vi "PID_controller_14.vi"() -> ()   [LabVIEW 2011]
panel:
  in  "Tune":bool
  out "Temp Set Point (torr)":dbl
  in  "stop":bool
  out "fit":cluster{"element":dbl, "Value":dbl}[](array[cluster])
  out "err_avg":dbl
  out "Setpoint":string
  in  "Ks":dbl
  out "dt(s)":dbl
  out "windup error":dbl
  out "tPrev":dbl
  out "target value":dbl
  out "error(t-t0)":cluster{dbl, "Value":dbl}[](array[cluster])
  out "error":dbl
  out "tStart(s)":dbl
  out "S00":dbl
  out "S10":dbl
  out "S20":dbl
  out "S11":dbl
  out "S01":dbl
  out "weight":dbl[](array[numeric])
  in  "# of points to watch":i32
  in  "tSmooth(s)":dbl=-1.0
  out "t0":dbl
  out "error(t)":cluster{dbl, "Value":dbl}[](array[cluster])
  out "error out":errorcluster
  out "first":bool=TRUE
  out "XY Graph":T1(graph)
  out "current value":dbl
  in  "Period (s)":dbl
  out "dValue":dbl
  out "derivative":dbl
  out "integral":dbl
  out "Angle (deg)":dbl
  in  "Kd":dbl
  in  "Ki":dbl
  in  "Kp":dbl
  out "Current P (torr)":dbl
  in  "Set Point (torr)":dbl
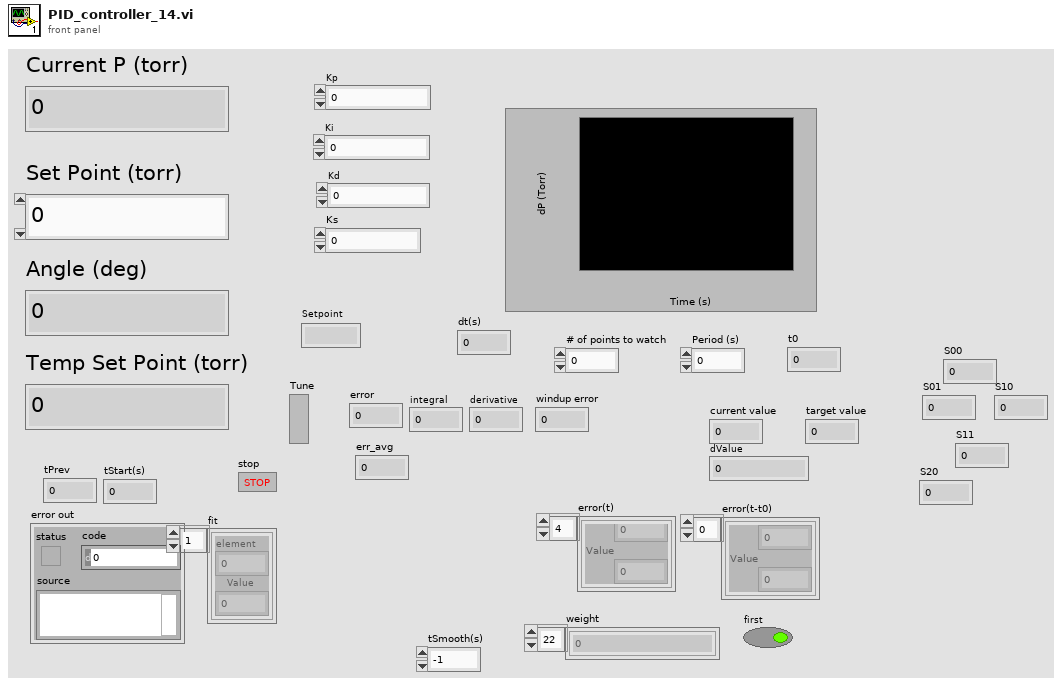
[diagram p1: front panel]
types:
  T1 = cluster{"Value":cluster{"element":dbl, "Value":dbl}[]}[]
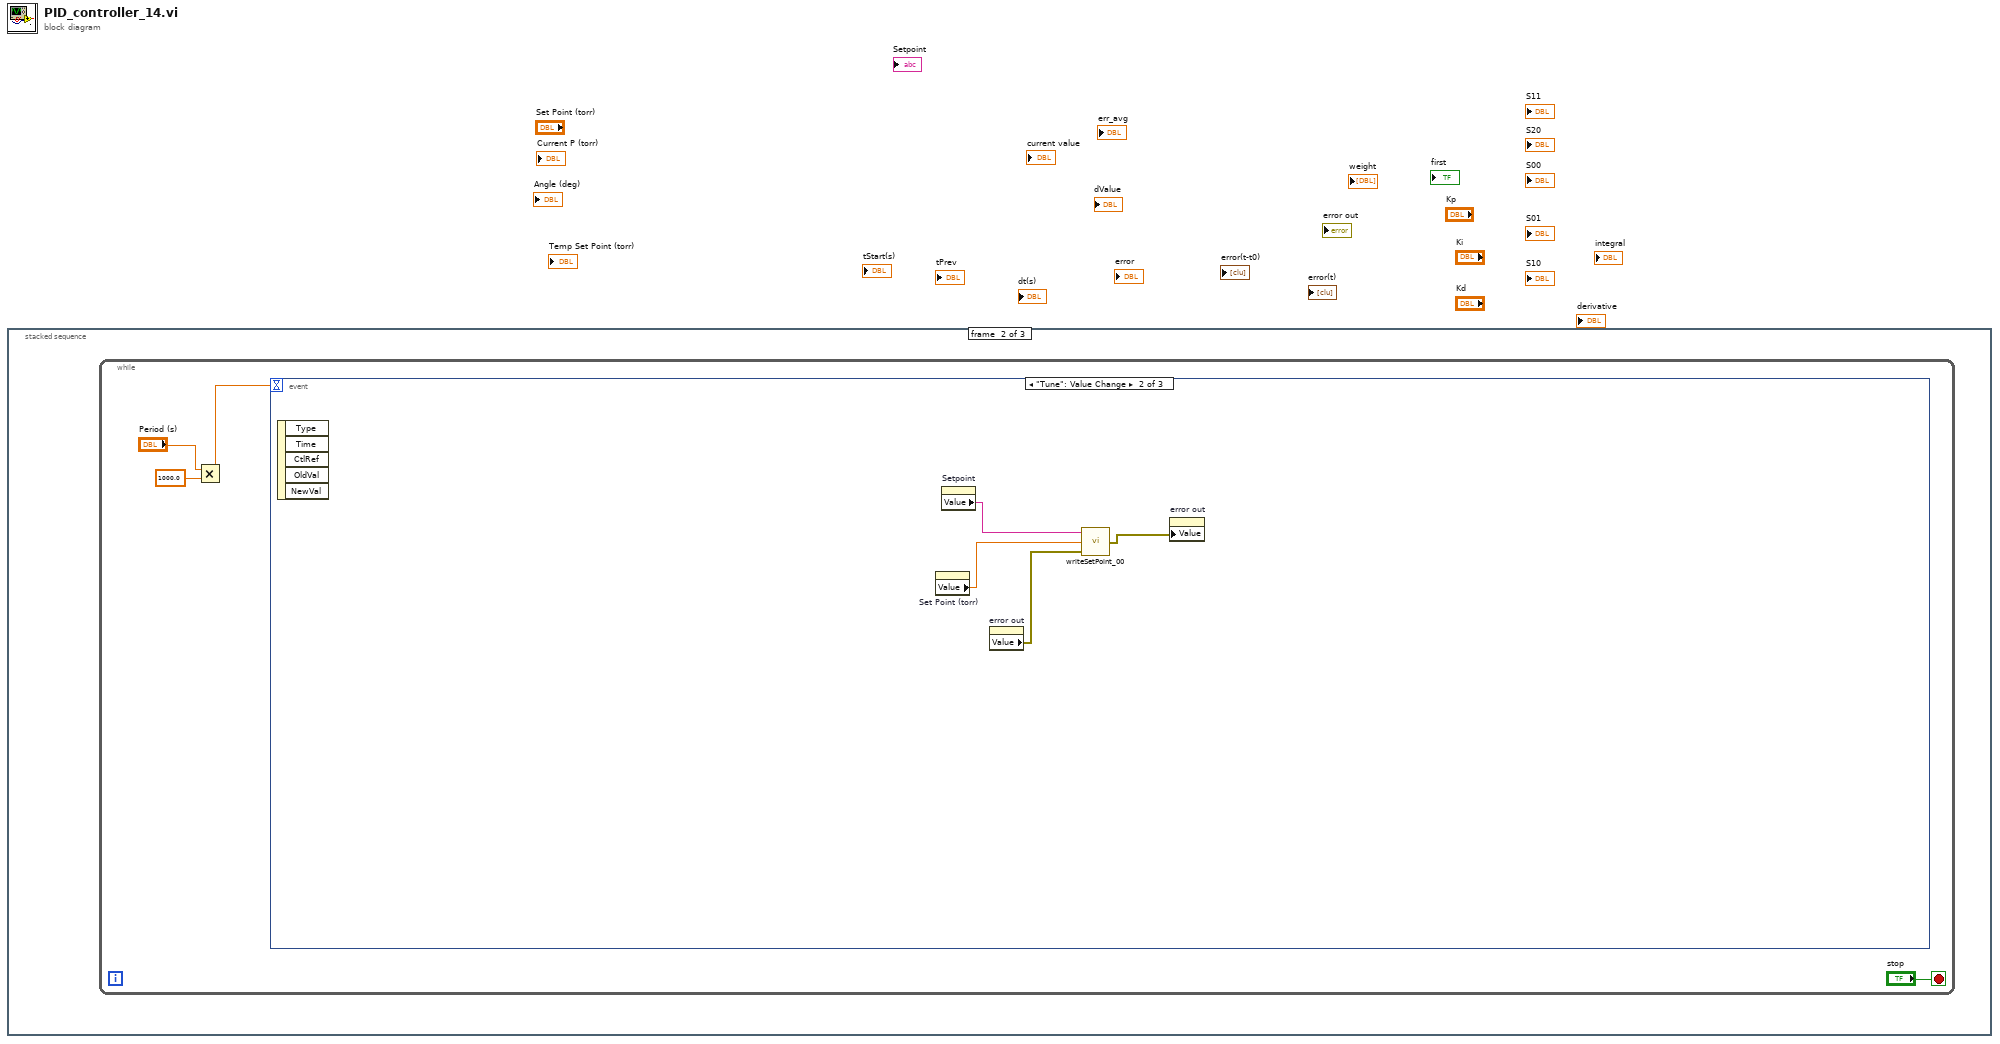
[diagram p0: block diagram]
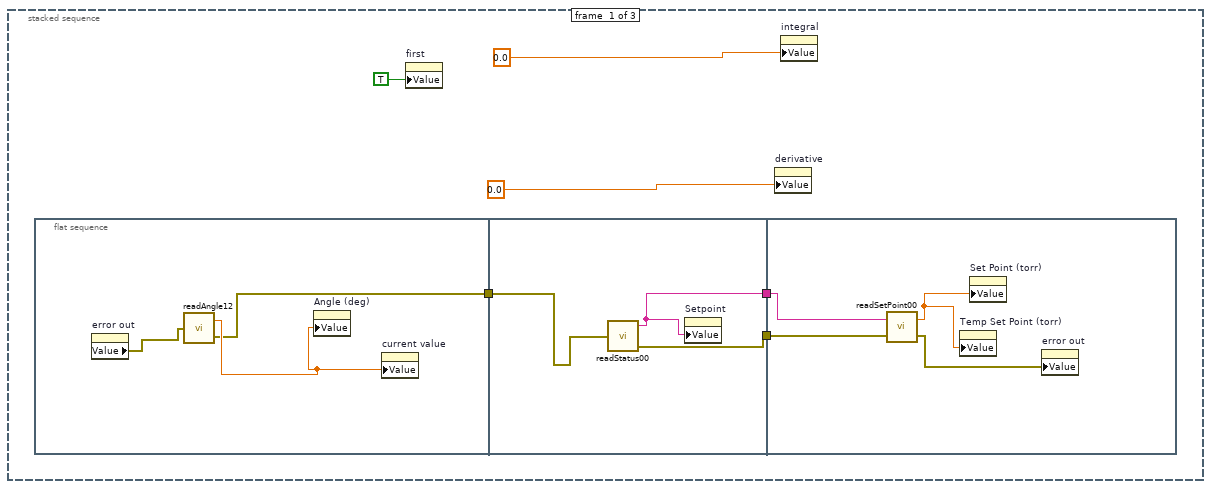
[diagram p2: hidden frame]
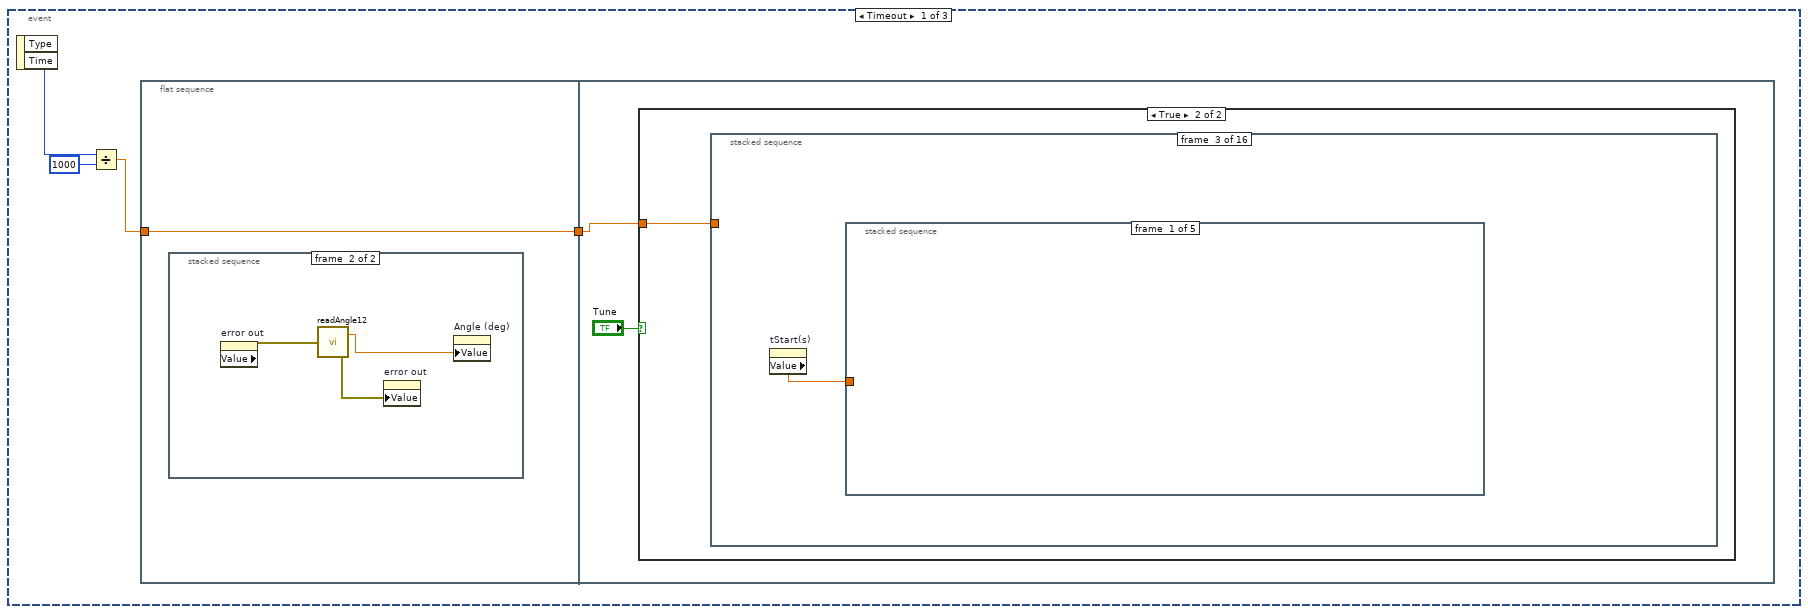
[diagram p3: hidden frame]
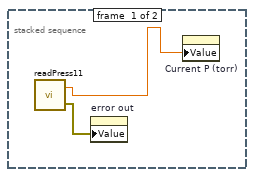
[diagram p4: hidden frame]
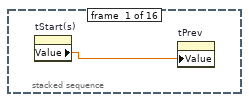
[diagram p6: hidden frame]
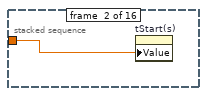
[diagram p7: hidden frame]
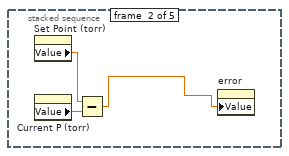
[diagram p8: hidden frame]
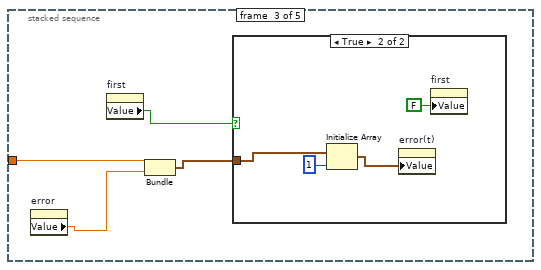
[diagram p9: hidden frame]
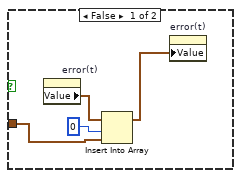
[diagram p10: hidden frame]
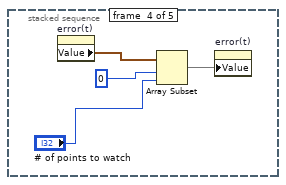
[diagram p11: hidden frame]
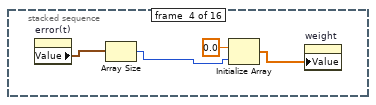
[diagram p13: hidden frame]
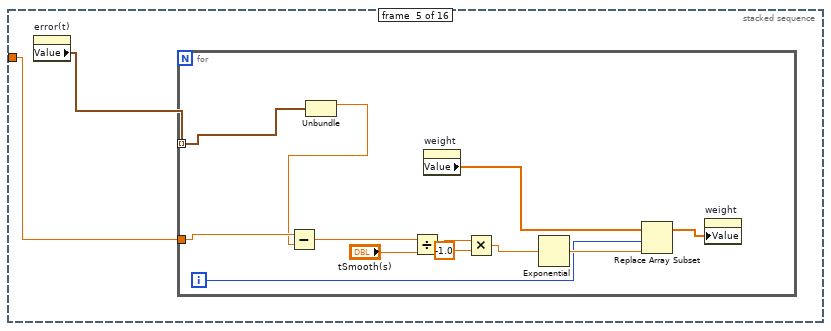
[diagram p14: hidden frame]
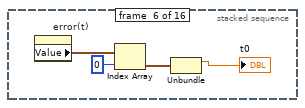
[diagram p15: hidden frame]
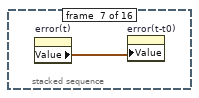
[diagram p16: hidden frame]
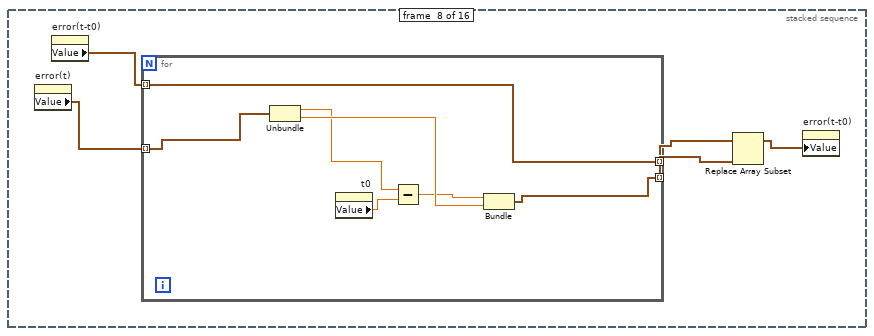
[diagram p17: hidden frame]
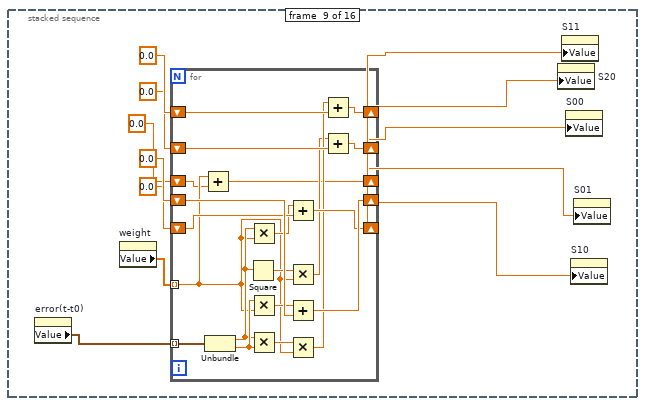
[diagram p18: hidden frame]
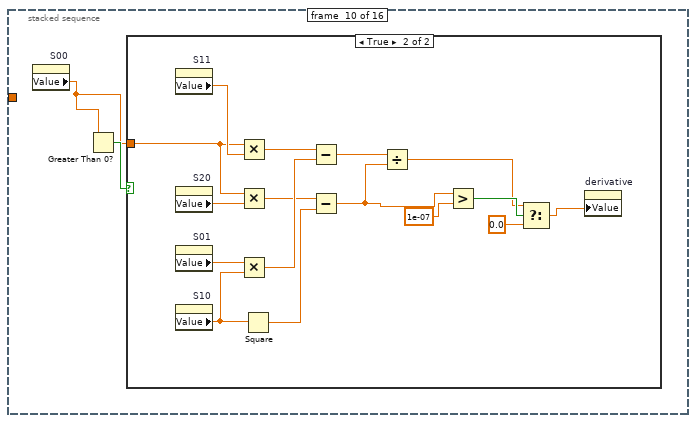
[diagram p19: hidden frame]
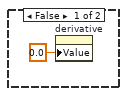
[diagram p20: hidden frame]
diagram:
  n1 = stacked-sequence {
    frame #0 {
      n2 = flat-sequence {
        tunnel: [w7] -> w1
        tunnel: [w10] -> w3
        tunnel: [w12] -> w2
        tunnel: w1 -> [w11]
        tunnel: w3 -> [w16]
        tunnel: w2 -> [w15]
        frame #0 {
          n3 = property on="error out" class="Clust (strict)"() -> ("Value"=w9:errorcluster)  [unwired: 2 in, 2 out]
          n4 = call "readAngle12.vi"("error in"=w9) -> ("angle"=w8:dbl, "error out"=w7:errorcluster)
          n5 = property on="Angle (deg)" class="DigNum (strict)"("Value"=w8) -> ()  [unwired: 2 in, 2 out]
          n6 = property on="current value" class="DigNum (strict)"("Value"=w8) -> ()  [unwired: 2 in, 2 out]
        }
        frame #1 {
          n7 = call "readStatus00.vi"("error in"=w11) -> ("Setpoint"=w10:string, "error out"=w12:errorcluster)  [unwired: 1 out]
          n8 = property on="Setpoint" class="Str"("Value"=w10) -> ()  [unwired: 2 in, 2 out]
        }
        frame #2 {
          n9 = call "readSetPoint00.vi"("error in"=w15, "Setpoint"=w16) -> ("error out"=w14:errorcluster, "P"=w13:dbl)
          n10 = property on="Temp Set Point (torr)" class="DigNum (strict)"("Value"=w13) -> ()  [unwired: 2 in, 2 out]
          n11 = property on="Set Point (torr)" class="DigNum (strict)"("Value"=w13) -> ()  [unwired: 2 in, 2 out]
          n12 = property on="error out" class="Clust (strict)"("Value"=w14) -> ()  [unwired: 2 in, 2 out]
        }
      }
      n13 = property on="first" class="Bool (strict)"("Value"=TRUE ("first")) -> ()  [unwired: 2 in, 2 out]
      n14 = property on="derivative" class="DigNum (strict)"("Value"=0.0 ("derivative")) -> ()  [unwired: 2 in, 2 out]
      n15 = property on="integral" class="DigNum (strict)"("Value"=0.0 ("integral")) -> ()  [unwired: 2 in, 2 out]
    }
    frame #1 {
      n16 = while {
        stop <- "stop" stop-if-true
        n17 = Multiply(x="Period (s)", y=1000.0) -> (x*y=w18:dbl)
        n18 = event shown="[1] \"Tune\": Value Change" {
          selector: _ -> [_ _ _]
          dyn-events: _ -> [_ _ _]
          timeout: w18 -> [_ _ _]
          event Timeout {
            n19 = event-data() -> ("Time"=w24:u32)  [unwired: 1 in, 1 out]
            n20 = Divide(x=w24, y=u32 1000) -> (x/y=w22:dbl)
            n21 = flat-sequence {
              tunnel: w22 -> [w25]
              tunnel: [w25] -> w21
              tunnel: w21 -> [w32]
              frame #0 {
                n22 = stacked-sequence {
                  frame #0 {
                    n23 = call "readPress11.vi"() -> ("P"=w27:dbl, "error out"=w26:errorcluster)  [unwired: 1 in]
                    n24 = property on="error out" class="Clust (strict)"("Value"=w26) -> ()  [unwired: 2 in, 2 out]
                    n25 = property on="Current P (torr)" class="DigNum (strict)"("Value"=w27) -> ()  [unwired: 2 in, 2 out]
                  }
                  frame #1 {
                    n26 = property on="error out" class="Clust (strict)"() -> ("Value"=w29:errorcluster)  [unwired: 2 in, 2 out]
                    n27 = call "readAngle12.vi"("error in"=w29) -> ("angle"=w30:dbl, "error out"=w28:errorcluster)
                    n28 = property on="error out" class="Clust (strict)"("Value"=w28) -> ()  [unwired: 2 in, 2 out]
                    n29 = property on="Angle (deg)" class="DigNum (strict)"("Value"=w30) -> ()  [unwired: 2 in, 2 out]
                  }
                }
              }
              frame #1 {
                n30 = case shown="True" "Tune" {
                  tunnel: w32 -> [_ w33]
                  frame False {
                  }
                  frame True {
                    n31 = stacked-sequence {
                      tunnel: w33 -> [_ w35 _ _ w60 _ _ _ _ _ _ _ _ _ _ _]
                      frame #0 {
                        n32 = property on="tStart(s)" class="DigNum (strict)"() -> ("Value"=w34:dbl)  [unwired: 2 in, 2 out]
                        n33 = property on="tPrev" class="DigNum (strict)"("Value"=w34) -> ()  [unwired: 2 in, 2 out]
                      }
                      frame #1 {
                        n34 = property on="tStart(s)" class="DigNum (strict)"("Value"=w35) -> ()  [unwired: 2 in, 2 out]
                      }
                      frame #2 {
                        n35 = property on="tStart(s)" class="DigNum (strict)"() -> ("Value"=w36:dbl)  [unwired: 2 in, 2 out]
                        n36 = stacked-sequence {
                          tunnel: w36 -> [_ _ w42 _ _]
                          frame #0 {
                          }
                          frame #1 {
                            n37 = property on="Set Point (torr)" class="DigNum (strict)"() -> ("Value"=w38:dbl)  [unwired: 2 in, 2 out]
                            n38 = property on="Current P (torr)" class="DigNum (strict)"() -> ("Value"=w39:dbl)  [unwired: 2 in, 2 out]
                            n39 = Subtract(x=w38, y=w39) -> (x-y=w37:dbl)
                            n40 = property on="error" class="DigNum (strict)"("Value"=w37) -> ()  [unwired: 2 in, 2 out]
                          }
                          frame #2 {
                            n41 = property on="error" class="DigNum (strict)"() -> ("Value"=w40:dbl)  [unwired: 2 in, 2 out]
                            n42 = property on="first" class="Bool (strict)"() -> ("Value"=w43:bool)  [unwired: 2 in, 2 out]
                            n43 = Bundle("Value"=w42, "Value"=w40) -> (w41:cluster{"Value":dbl, "Value":dbl})  [unwired: 1 in]
                            n44 = case shown="True" w43 {
                              tunnel: w41 -> [w45 w50]
                              frame False {
                                n45 = property on="error(t)" class="Arr (strict)"() -> ("Value"=w46:cluster{dbl, "Value":dbl}[])  [unwired: 2 in, 2 out]
                                n46 = Insert Into Array(array=w46, index=0, new element=w45) -> (w44:cluster{dbl, "Value":dbl}[])
                                n47 = property on="error(t)" class="Arr (strict)"("Value"=w44) -> ()  [unwired: 2 in, 2 out]
                              }
                              frame True {
                                n48 = Initialize Array(w50, 1 ("dimension size")) -> (w48:cluster{"Value":dbl, "Value":dbl}[])
                                n49 = property on="error(t)" class="Arr (strict)"("Value"=w48) -> ()  [unwired: 2 in, 2 out]
                                n50 = property on="first" class="Bool (strict)"("Value"=FALSE ("first")) -> ()  [unwired: 2 in, 2 out]
                              }
                            }
                          }
                          frame #3 {
                            n51 = property on="error(t)" class="Arr (strict)"() -> ("Value"=w53:cluster{dbl, "Value":dbl}[])  [unwired: 2 in, 2 out]
                            n52 = Array Subset(array=w53, index=0, length="# of points to watch") -> (w55:cluster{dbl, "Value":dbl}[])
                            n53 = property on="error(t)" class="Arr (strict)"("Value"=w55) -> ()  [unwired: 2 in, 2 out]
                          }
                          frame #4 {
                          }
                        }
                      }
                      frame #3 {
                        n54 = property on="error(t)" class="Arr (strict)"() -> ("Value"=w59:cluster{dbl, "Value":dbl}[])  [unwired: 2 in, 2 out]
                        n55 = Array Size(array=w59) -> (size(s)=w57:i32)
                        n56 = Initialize Array(0.0 ("element"), w57) -> (w56:dbl[])
                        n57 = property on="weight" class="Arr (strict)"("Value"=w56) -> ()  [unwired: 2 in, 2 out]
                      }
                      frame #4 {
                        n58 = property on="error(t)" class="Arr (strict)"() -> ("Value"=w61:cluster{dbl, "Value":dbl}[])  [unwired: 2 in, 2 out]
                        n59 = for {
                          tunnel: w61 -> [w73] mode=indexing
                          tunnel: w60 -> [w72]
                          i -> [w68]
                          n60 = Unbundle(w73) -> (w71:dbl)  [unwired: 1 out]
                          n61 = Subtract(x=w72, y=w71) -> (x-y=w66:dbl)
                          n62 = Divide(x=w66, y="tSmooth(s)") -> (x/y=w64:dbl)
                          n63 = property on="weight" class="Arr (strict)"() -> ("Value"=w69:dbl[])  [unwired: 2 in, 2 out]
                          n64 = Multiply(x=w64, y=-1.0) -> (x*y=w62:dbl)
                          n65 = Exponential(1:w62) -> (0:w70:dbl)
                          n66 = Replace Array Subset(array=w69, new element=w70, index=w68) -> (w67:dbl[])
                          n67 = property on="weight" class="Arr (strict)"("Value"=w67) -> ()  [unwired: 2 in, 2 out]
                        }
                      }
                      frame #5 {
                        n68 = property on="error(t)" class="Arr (strict)"() -> ("Value"=w77:cluster{dbl, "Value":dbl}[])  [unwired: 2 in, 2 out]
                        n69 = Index Array(array=w77, index=0) -> (element=w75:cluster{dbl, "Value":dbl})
                        n70 = Unbundle(w75) -> (→"t0":dbl)  [unwired: 1 out]
                      }
                      frame #6 {
                        n71 = property on="error(t)" class="Arr (strict)"() -> ("Value"=w78:cluster{dbl, "Value":dbl}[])  [unwired: 2 in, 2 out]
                        n72 = property on="error(t-t0)" class="Arr (strict)"("Value"=w78) -> ()  [unwired: 2 in, 2 out]
                      }
                      frame #7 {
                        n73 = property on="error(t)" class="Arr (strict)"() -> ("Value"=w83:cluster{dbl, "Value":dbl}[])  [unwired: 2 in, 2 out]
                        n74 = property on="error(t-t0)" class="Arr (strict)"() -> ("Value"=w81:cluster{dbl, "Value":dbl}[])  [unwired: 2 in, 2 out]
                        n75 = for {
                          tunnel: w83 -> [w86] mode=indexing
                          tunnel: [w85] -> w82 mode=indexing
                          tunnel: w81 -> [w84] mode=indexing
                          tunnel: [w84] -> w80 mode=indexing
                          n76 = Unbundle(w86) -> (w87:dbl, "Value"=w89:dbl)
                          n77 = property on="t0" class="DigNum (strict)"() -> ("Value"=w90:dbl)  [unwired: 2 in, 2 out]
                          n78 = Subtract(x=w87, y=w90) -> (x-y=w88:dbl)
                          n79 = Bundle(w88, "Value"=w89) -> (w85:cluster{dbl, "Value":dbl})  [unwired: 1 in]
                        }
                        n80 = Replace Array Subset(array=w80, new element=w82) -> (w79:cluster{dbl, "Value":dbl}[])  [unwired: 1 in]
                        n81 = property on="error(t-t0)" class="Arr (strict)"("Value"=w79) -> ()  [unwired: 2 in, 2 out]
                      }
                      frame #8 {
                        n82 = property on="error(t-t0)" class="Arr (strict)"() -> ("Value"=w91:cluster{dbl, "Value":dbl}[])  [unwired: 2 in, 2 out]
                        n83 = property on="weight" class="Arr (strict)"() -> ("Value"=w98:dbl[])  [unwired: 2 in, 2 out]
                        n84 = for {
                          tunnel: w91 -> [w118] mode=indexing
                          shift-right: [w119] -> w93
                          shift-left: 0.0 -> [w122]
                          shift-right: [w115] -> w96
                          shift-left: 0.0 -> [w121]
                          shift-right: [w114] -> w95
                          shift-left: 0.0 -> [w120]
                          shift-right: [w116] -> w92
                          shift-left: 0.0 -> [w117]
                          tunnel: w98 -> [w105] mode=indexing
                          shift-right: [w103] -> w94
                          shift-left: 0.0 -> [w104]
                          n85 = Add(x=w105, y=w104) -> (x+y=w103:dbl)
                          n86 = Unbundle(w118) -> (w107:dbl, "Value"=w113:dbl)
                          n87 = Square(x=w107) -> (x^2=w109:dbl)
                          n88 = Multiply(x=w107, y=w105) -> (x*y=w106:dbl)
                          n89 = Multiply(x=w113, y=w105) -> (x*y=w112:dbl)
                          n90 = Multiply(x=w107, y=w113) -> (x*y=w111:dbl)
                          n91 = Add(x=w106, y=w117) -> (x+y=w116:dbl)
                          n92 = Multiply(x=w109, y=w105) -> (x*y=w108:dbl)
                          n93 = Add(x=w112, y=w122) -> (x+y=w119:dbl)
                          n94 = Multiply(x=w111, y=w105) -> (x*y=w110:dbl)
                          n95 = Add(x=w110, y=w121) -> (x+y=w115:dbl)
                          n96 = Add(x=w108, y=w120) -> (x+y=w114:dbl)
                        }
                        n97 = property on="S20" class="DigNum (strict)"("Value"=w95) -> ()  [unwired: 2 in, 2 out]
                        n98 = property on="S11" class="DigNum (strict)"("Value"=w96) -> ()  [unwired: 2 in, 2 out]
                        n99 = property on="S00" class="DigNum (strict)"("Value"=w94) -> ()  [unwired: 2 in, 2 out]
                        n100 = property on="S10" class="DigNum (strict)"("Value"=w92) -> ()  [unwired: 2 in, 2 out]
                        n101 = property on="S01" class="DigNum (strict)"("Value"=w93) -> ()  [unwired: 2 in, 2 out]
                      }
                      frame #9 {
                        n102 = property on="S00" class="DigNum (strict)"() -> ("Value"=w123:dbl)  [unwired: 2 in, 2 out]
                        n103 = Greater Than 0?(x=w123) -> (x > 0?=w124:bool)
                        n104 = case shown="True" w124 {
                          tunnel: w123 -> [_ w133]
                          frame False {
                            n105 = property on="derivative" class="DigNum (strict)"("Value"=0.0 ("derivative")) -> ()  [unwired: 2 in, 2 out]
                          }
                          frame True {
                            n106 = property on="S11" class="DigNum (strict)"() -> ("Value"=w135:dbl)  [unwired: 2 in, 2 out]
                            n107 = property on="S20" class="DigNum (strict)"() -> ("Value"=w134:dbl)  [unwired: 2 in, 2 out]
                            n108 = property on="S01" class="DigNum (strict)"() -> ("Value"=w132:dbl)  [unwired: 2 in, 2 out]
                            n109 = property on="S10" class="DigNum (strict)"() -> ("Value"=w136:dbl)  [unwired: 2 in, 2 out]
                            n110 = Multiply(x=w133, y=w135) -> (x*y=w141:dbl)
                            n111 = Multiply(x=w133, y=w134) -> (x*y=w139:dbl)
                            n112 = Multiply(x=w132, y=w136) -> (x*y=w140:dbl)
                            n113 = Square(x=w136) -> (x^2=w138:dbl)
                            n114 = Subtract(x=w141, y=w140) -> (x-y=w137:dbl)
                            n115 = Subtract(x=w139, y=w138) -> (x-y=w131:dbl)
                            n116 = Divide(x=w137, y=w131) -> (x/y=w127:dbl)
                            n117 = Greater?(x=w131, y=1e-07) -> (0:w129:bool)
                            n118 = Select(t=w127, s=w129, f=0.0) -> (s? t:f=w128:dbl)
                            n119 = property on="derivative" class="DigNum (strict)"("Value"=w128) -> ()  [unwired: 2 in, 2 out]
                          }
                        }
                      }
                      frame #10 {
                        n120 = property on="S00" class="DigNum (strict)"() -> ("Value"=w142:dbl)  [unwired: 2 in, 2 out]
                        n121 = Greater Than 0?(x=w142) -> (x > 0?=w143:bool)
                        n122 = case shown="True" w143 {
                          tunnel: w142 -> [_ w146]
                          frame False {
                            n123 = property on="err_avg" class="DigNum (strict)"("Value"=0.0 ("Pavg")) -> ()  [unwired: 2 in, 2 out]
                          }
                          frame True {
                            n124 = property on="S01" class="DigNum (strict)"() -> ("Value"=w147:dbl)  [unwired: 2 in, 2 out]
                            n125 = property on="S20" class="DigNum (strict)"() -> ("Value"=w150:dbl)  [unwired: 2 in, 2 out]
                            n126 = property on="S11" class="DigNum (strict)"() -> ("Value"=w148:dbl)  [unwired: 2 in, 2 out]
                            n127 = property on="S11" class="DigNum (strict)"() -> ("Value"=w149:dbl)  [unwired: 2 in, 2 out]
                            n128 = Multiply(x=w147, y=w150) -> (x*y=w155:dbl)
                            n129 = Multiply(x=w146, y=w150) -> (x*y=w152:dbl)
                            n130 = Multiply(x=w149, y=w148) -> (x*y=w156:dbl)
                            n131 = Square(x=w149) -> (x^2=w153:dbl)
                            n132 = Subtract(x=w155, y=w156) -> (x-y=w151:dbl)
                            n133 = Subtract(x=w152, y=w153) -> (x-y=w154:dbl)
                            n134 = Divide(x=w151, y=w154) -> (x/y=w145:dbl)
                            n135 = property on="err_avg" class="DigNum (strict)"("Value"=w145) -> ()  [unwired: 2 in, 2 out]
                          }
                        }
                      }
                      frame #11 {
                        n136 = property on="error(t-t0)" class="Arr (strict)"() -> ("Value"=w160:cluster{dbl, "Value":dbl}[])  [unwired: 2 in, 2 out]
                        n137 = Array Size(array=w160) -> (size(s)=w159:i32)
                        n138 = Greater?(x=w159, y=1) -> (0:w157:bool)
                        n139 = case shown="True" w157 {
                          frame False {
                          }
                          frame True {
                            n140 = property on="error(t-t0)" class="Arr (strict)"() -> ("Value"=w164:cluster{dbl, "Value":dbl}[])  [unwired: 2 in, 2 out]
                            n141 = Array Size(array=w164) -> (size(s)=w174:i32)
                            n142 = Index Array(array=w164, index=0) -> (element=w172:cluster{dbl, "Value":dbl})
                            n143 = Unbundle(w172) -> (w167:dbl)  [unwired: 1 out]
                            n144 = Decrement(x=w174) -> (x-1=w173:i32)
                            n145 = Index Array(array=w164, index=w173) -> (element=w171:cluster{dbl, "Value":dbl})
                            n146 = Unbundle(w171) -> (w165:dbl)  [unwired: 1 out]
                            n147 = property on="derivative" class="DigNum (strict)"() -> ("Value"=w170:dbl)  [unwired: 2 in, 2 out]
                            n148 = property on="error" class="DigNum (strict)"() -> ("Value"=w168:dbl)  [unwired: 2 in, 2 out]
                            n149 = Multiply(x=w165, y=w170) -> (x*y=w169:dbl)
                            n150 = Add(x=w168, y=w169) -> (x+y=w166:dbl)
                            n151 = Bundle(w167, "Value"=w168) -> (w163:cluster{dbl, "Value":dbl})  [unwired: 1 in]
                            n152 = Bundle(w165, w166) -> (w162:cluster{dbl, dbl})  [unwired: 1 in]
                            n153 = Build Array(w163, w162) -> (→"fit":cluster{dbl, "Value":dbl}[])
                          }
                        }
                      }
                      frame #12 {
                        n154 = property on="error" class="DigNum (strict)"() -> ("Value"=w180:dbl)  [unwired: 2 in, 2 out]
                        n155 = property on="tPrev" class="DigNum (strict)"() -> ("Value"=w181:dbl)  [unwired: 2 in, 2 out]
                        n156 = property on="tStart(s)" class="DigNum (strict)"() -> ("Value"=w182:dbl)  [unwired: 2 in, 2 out]
                        n157 = Subtract(x=w182, y=w181) -> (x-y=w176:dbl)
                        n158 = property on="dt(s)" class="DigNum (strict)"("Value"=w176) -> ()  [unwired: 2 in, 2 out]
                        n159 = property on="integral" class="DigNum (strict)"() -> ("Value"=w178:dbl)  [unwired: 2 in, 2 out]
                        n160 = Multiply(x=w180, y=w176) -> (x*y=w179:dbl)
                        n161 = Add(x=w179, y=w178) -> (x+y=w177:dbl)
                        n162 = property on="integral" class="DigNum (strict)"("Value"=w177) -> ()  [unwired: 2 in, 2 out]
                      }
                      frame #13 {
                        n163 = property on="error" class="DigNum (strict)"() -> ("Value"=w183:dbl)  [unwired: 2 in, 2 out]
                        n164 = property on="Kp" class="DigNum (strict)"() -> ("Value"=w193:dbl)  [unwired: 2 in, 2 out]
                        n165 = property on="integral" class="DigNum (strict)"() -> ("Value"=w191:dbl)  [unwired: 2 in, 2 out]
                        n166 = property on="derivative" class="DigNum (strict)"() -> ("Value"=w189:dbl)  [unwired: 2 in, 2 out]
                        n167 = property on="Ki" class="DigNum (strict)"() -> ("Value"=w192:dbl)  [unwired: 2 in, 2 out]
                        n168 = property on="Kd" class="DigNum (strict)"() -> ("Value"=w190:dbl)  [unwired: 2 in, 2 out]
                        n169 = Multiply(x=w190, y=w189) -> (x*y=w186:dbl)
                        n170 = Multiply(x=w192, y=w191) -> (x*y=w187:dbl)
                        n171 = Multiply(x=w193, y=w183) -> (x*y=w188:dbl)
                        n172 = Add(x=w188, y=w187) -> (x+y=w185:dbl)
                        n173 = Add(x=w185, y=w186) -> (x+y=w184:dbl)
                        n174 = property on="dValue" class="DigNum (strict)"("Value"=w184) -> ()  [unwired: 2 in, 2 out]
                      }
                      frame #14 {
                        w204 = 90.0 ("y")
                        n175 = property on="dValue" class="DigNum (strict)"() -> ("Value"=w211:dbl)  [unwired: 2 in, 2 out]
                        n176 = property on="current value" class="DigNum (strict)"() -> ("Value"=w212:dbl)  [unwired: 2 in, 2 out]
                        n177 = Add(x=w212, y=w211) -> (x+y=w196:dbl)
                        "target value" <- w196
                        n178 = Less Than 0?(x=w196) -> (x < 0?=w208:bool)
                        n179 = Select(t=0.0, s=w208, f=w196) -> (s? t:f=w205:dbl)
                        n180 = property on="Setpoint" class="Str"() -> ("Value"=w195:string)  [unwired: 2 in, 2 out]
                        n181 = property on="error out" class="Clust (strict)"() -> ("Value"=w210:errorcluster)  [unwired: 2 in, 2 out]
                        n182 = Greater?(x=w205, y=w204) -> (0:w206:bool)
                        n183 = Select(t=w204, s=w206, f=w205) -> (s? t:f=w194:dbl)
                        n184 = Subtract(x=w194, y=w196) -> (x-y=w203:dbl)
                        "windup error" <- w203
                        n185 = call "writeSetPoint_00.vi"("error in"=w210, "P (Torr)"=w194, "Setpoint"=w195) -> ("error out"=w209:errorcluster)
                        n186 = property on="dt(s)" class="DigNum (strict)"() -> ("Value"=w202:dbl)  [unwired: 2 in, 2 out]
                        n187 = property on="Temp Set Point (torr)" class="DigNum (strict)"("Value"=w194) -> ()  [unwired: 2 in, 2 out]
                        n188 = property on="current value" class="DigNum (strict)"("Value"=w194) -> ()  [unwired: 2 in, 2 out]
                        n189 = property on="error out" class="Clust (strict)"("Value"=w209) -> ()  [unwired: 2 in, 2 out]
                        n190 = Multiply(x=w203, y=w202) -> (x*y=w201:dbl)
                        n191 = property on="integral" class="DigNum (strict)"() -> ("Value"=w198:dbl)  [unwired: 2 in, 2 out]
                        n192 = Multiply(x="Ks", y=w201) -> (x*y=w199:dbl)
                        n193 = Add(x=w199, y=w198) -> (x+y=w197:dbl)
                        n194 = property on="integral" class="DigNum (strict)"("Value"=w197) -> ()  [unwired: 2 in, 2 out]
                      }
                      frame #15 {
                        n195 = property on="fit" class="Arr (strict)"() -> ("Value"=w215:cluster{"element":dbl, "Value":dbl}[])  [unwired: 2 in, 2 out]
                        n196 = property on="error(t-t0)" class="Arr (strict)"() -> ("Value"=w214:cluster{dbl, "Value":dbl}[])  [unwired: 2 in, 2 out]
                        n197 = Build Cluster Array(w214, w215) -> (→"XY Graph":T1)
                      }
                    }
                  }
                }
              }
            }
          }
          event "Tune": Value Change {
            n198 = event-data() -> ()  [unwired: 1 in, 5 out]
            n199 = property on="Set Point (torr)" class="DigNum (strict)"() -> ("Value"=w218:dbl)  [unwired: 2 in, 2 out]
            n200 = property on="Setpoint" class="Str"() -> ("Value"=w219:string)  [unwired: 2 in, 2 out]
            n201 = property on="error out" class="Clust (strict)"() -> ("Value"=w217:errorcluster)  [unwired: 2 in, 2 out]
            n202 = call "writeSetPoint_00.vi"("error in"=w217, "P (Torr)"=w218, "Setpoint"=w219) -> ("error out"=w216:errorcluster)
            n203 = property on="error out" class="Clust (strict)"("Value"=w216) -> ()  [unwired: 2 in, 2 out]
          }
          event "Set Point (torr)": Value Change {
            n204 = event-data() -> ()  [unwired: 1 in, 5 out]
            n205 = property on="Set Point (torr)" class="DigNum (strict)"() -> ("Value"=w222:dbl)  [unwired: 2 in, 2 out]
            n206 = property on="Setpoint" class="Str"() -> ("Value"=w223:string)  [unwired: 2 in, 2 out]
            n207 = property on="error out" class="Clust (strict)"() -> ("Value"=w221:errorcluster)  [unwired: 2 in, 2 out]
            n208 = call "writeSetPoint_00.vi"("error in"=w221, "P (Torr)"=w222, "Setpoint"=w223) -> ("error out"=w220:errorcluster)
            n209 = property on="error out" class="Clust (strict)"("Value"=w220) -> ()  [unwired: 2 in, 2 out]
          }
        }
      }
    }
    frame #2 {
      n210 = disable-structure shown="Disabled" {
        frame Disabled {
          n211 = flat-sequence {
            frame #0 {
              n212 = call "WriteAdaptorr03.vi"("string to write"="D5") -> ()  [unwired: 1 in, 1 out]
            }
            frame #1 {
              n213 = property on="Setpoint" class="Str"() -> ("Value"=w226:string)  [unwired: 2 in, 2 out]
              n214 = Concatenate Strings("Press ", w226, " on AdapTorr") -> (w225:string)
              n215 = One Button Dialog(message=w225) -> ()  [unwired: 1 in, 1 out]
            }
          }
        }
        frame Enabled {
        }
      }
    }
  }
